vi "ActuatorOutput.vi"(0 "FPGA VI Reference In":refnum<k20>, 1 "Cluster in":T1, 3 "error in (no error)":errorcluster) -> (7 "FPGA VI Reference Out":refnum<k20>, 8 "Cluster out":T1, 10 "error out":errorcluster)   [LabVIEW 2018]
uses:
  Type_Def/Type_Def Actuator Controls.ctl
  <vilib>/Utility/error.llb/Error Cluster From Error Code.vi
  <vilib>/rvi/errors/niLvFpgaAdjustHostInterfaceError.vi
  <vilib>/rvi/interface/nirviReadWriteControl/nirviReadWriteControl.xnode
  NiFpgaLv.dll
  <vilib>/rvi/interface/Simulation/niFpgaSimulationCallBeginRW.vi
panel:
  out "error out 2":errorcluster
  in  "error in":errorcluster
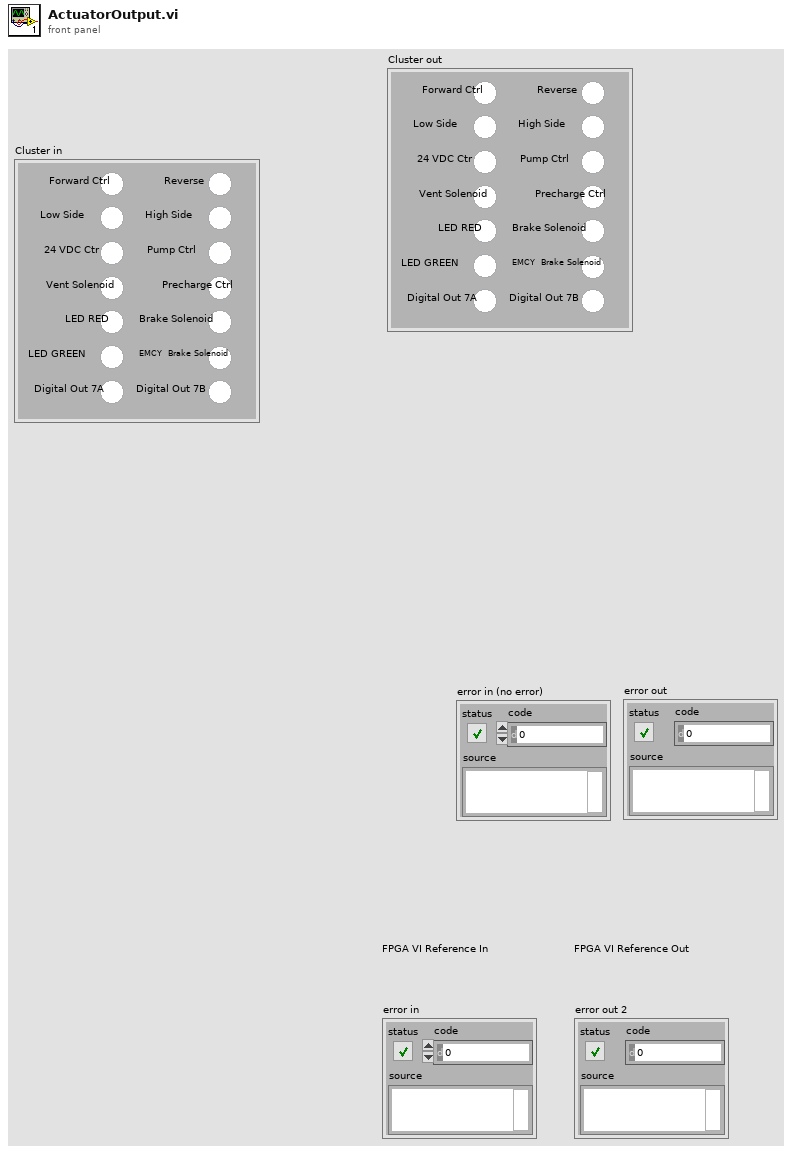
[diagram p1: front panel]
types:
  T1 = typedef "Type_Def Actuator Controls.ctl" = cluster{"Reverse ":bool, "Precharge Ctrl":bool, "Pump Ctrl":bool, "24 VDC Ctr":bool, "Vent Solenoid":bool, "Brake Solenoid":bool, "EMCY  Brake Solenoid":bool, "Digital Out 7B ":bool, "Forward Ctrl":bool, " Low Side":bool, "High Side":bool, "LED RED":bool, "LED GREEN":bool, " Digital Out 7A":bool}
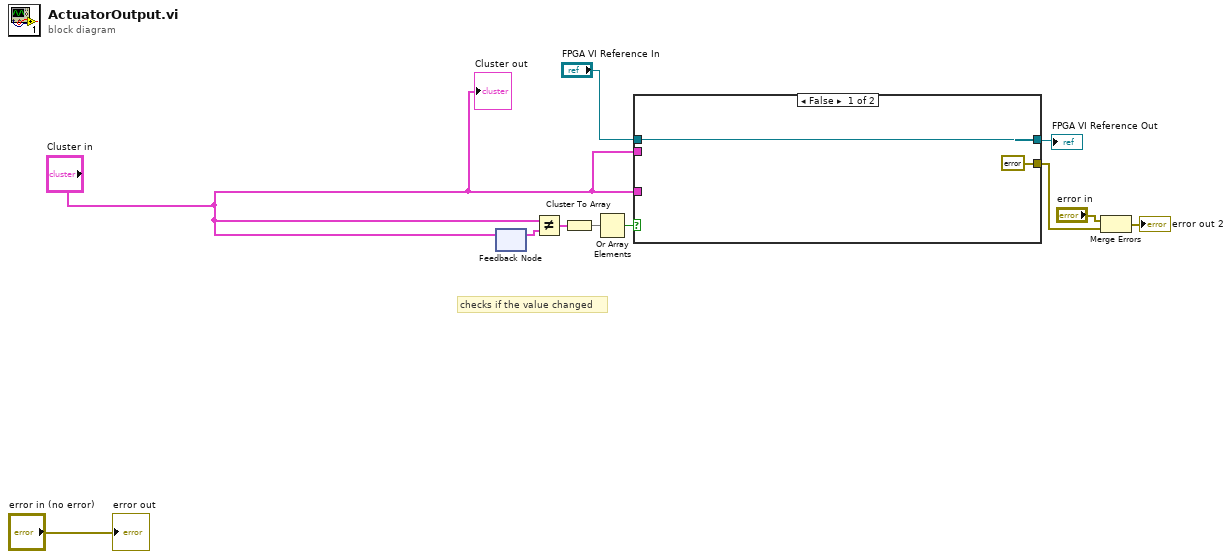
[diagram p0: block diagram]
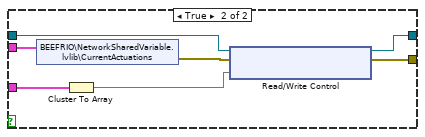
[diagram p2: hidden frame]
diagram:
  # "checks if the value changed"
  n1 = feedback #1() -> (w10:T1)  [unwired: 1 in]
  n2 = feedback-in #1("Cluster in") -> ()
  n3 = Not Equal?(x="Cluster in", y=w10) -> (x != y?=w8:T1)
  n4 = Cluster To Array(cluster=w8) -> (array=w7:bool[])
  n5 = Or Array Elements(Boolean array=w7) -> (logical OR=w9:bool)
  n6 = case shown="False" w9 {
    tunnel: [errorcluster {"status"=FALSE, "code"=0, "source"=""} ("error out") w20] -> w3
    tunnel: "Cluster in" -> [_ w14]
    tunnel: "FPGA VI Reference In" -> [w13 w18]
    tunnel: [w13 w19] -> w5
    tunnel: "Cluster in" -> [_ w15]
    frame False {
    }
    frame True {
      n7 = shared-variable "BEEFRIO\\NetworkSharedVariable.lvlib\\CurrentActuations"(w15) -> (error out=w17:errorcluster)  [unwired: 1 in]
      n8 = Cluster To Array(cluster=w14) -> (array=w16:bool[])
      n9 = xnode "Read/Write Control"("FPGA VI Reference In"=w18, "error in"=w17, "Digital Control Outputs"=w16) -> ("FPGA VI Reference Out"=w19:refnum<k20>, "error out"=w20:errorcluster)
    }
  }
  "FPGA VI Reference Out" <- w5
  n10 = Merge Errors("error in", w3) -> (→"error out 2":errorcluster)
  "error out" <- "error in (no error)"
  "Cluster out" <- "Cluster in"
